vi "setAttributeByName.vi"(8 "error in (no error)":errorcluster, 9 "attributeValue":string, 10 "attributeName":string, 11 "xmlNode in":refnum<class "xmlNode.lvclass">) -> (0 "error out":errorcluster, 3 "xmlNode out":refnum<class "xmlNode.lvclass">)   [LabVIEW 2011, in "Tools.lvlib" / "xml.lvlib" / "xmlNode.lvclass"]
uses:
  xmlNode.lvclass
  xmlNode.lvclass/xmlNode.ctl
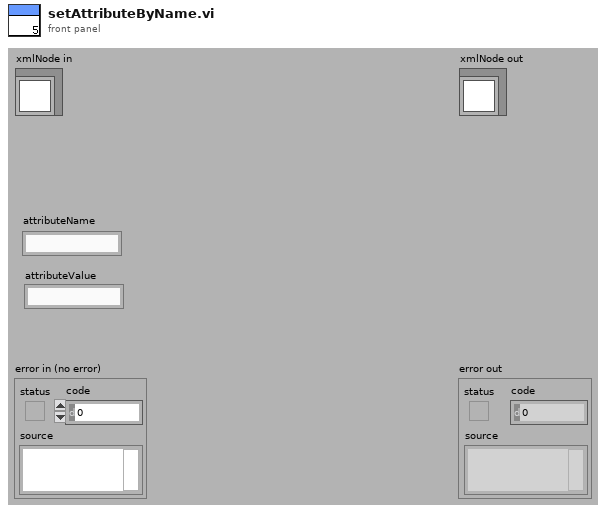
[diagram p1: front panel]
types:
  T1 = cluster{"attribute type":string, "attribute string":string}
  T2 = cluster{"attribute type":string, "attribute string":string}[]
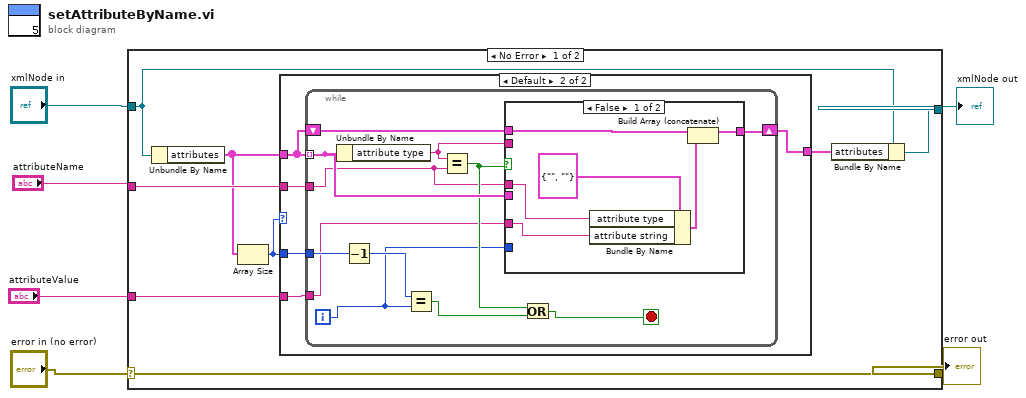
[diagram p0: block diagram]
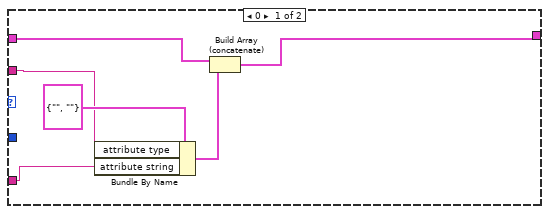
[diagram p2: hidden frame]
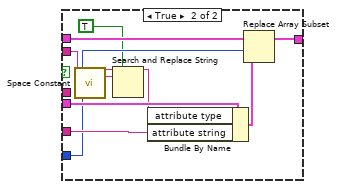
[diagram p3: hidden frame]
diagram:
  n1 = case shown="No Error" "error in (no error)" {
    selector: "error in (no error)" -> [w14 w55]
    tunnel: [w14 w55] -> w4
    tunnel: [w7 w54] -> w3
    tunnel: "xmlNode in" -> [w9 w54]
    tunnel: "attributeName" -> [w13 _]
    tunnel: "attributeValue" -> [w10 _]
    frame No Error {
      n2 = Unbundle By Name(w9) -> ("attributes"=w12:T2)
      n3 = Array Size(array=w12) -> (size(s)=w11:i32)
      n4 = case shown="Default" w11 {
        tunnel: w13 -> [w18 w25]
        tunnel: w12 -> [w16 w21]
        tunnel: w11 -> [_ w24]
        tunnel: [w15 w23] -> w8
        tunnel: w10 -> [w19 w22]
        frame 0 {
          n5 = Bundle By Name(cluster=T1 {"attribute type"="", "attribute string"=""} ("attribute"), "attribute type"=w18, "attribute string"=w19) -> (w17:T1)
          n6 = Build Array (concatenate)(w16, w17) -> (w15:T2)
        }
        frame Default {
          n7 = while {
            tunnel: w21 -> [w37] mode=indexing
            tunnel: w25 -> [w26]
            tunnel: w24 -> [w35]
            tunnel: w22 -> [w30]
            shift-right: [w28] -> w23
            shift-left: w21 -> [w29]
            i -> [w27]
            stop <- w32 stop-if-true
            n8 = Unbundle By Name(w37) -> ("attribute type"=w31:string)
            n9 = Decrement(x=w35) -> (x-1=w34:i32)
            n10 = Equal?(x=w34, y=w27) -> (x = y?=w33:bool)
            n11 = Equal?(x=w31, y=w26) -> (x = y?=w36:bool)
            n12 = case shown="False" w36 {
              tunnel: w37 -> [_ w53]
              tunnel: w31 -> [_ w47]
              tunnel: w30 -> [w39 w52]
              tunnel: w29 -> [w43 w51]
              tunnel: [w42 w50] -> w28
              tunnel: w27 -> [_ w48]
              tunnel: w26 -> [w40 _]
              frame False {
                n13 = Bundle By Name(cluster=T1 {"attribute type"="", "attribute string"=""} ("attribute"), "attribute type"=w40, "attribute string"=w39) -> (w38:T1)
                n14 = Build Array (concatenate)(w43, w38) -> (w42:T2)
              }
              frame True {
                n15 = call <vilib>:"Space Constant.vi"() -> ("String"=w44:string)
                n16 = Search and Replace String(replace all?=TRUE, input string=w47, search string=w44) -> (result string=w46:string)  [unwired: 5 in, 3 out]
                n17 = Bundle By Name(cluster=w53, "attribute type"=w46, "attribute string"=w52) -> (w49:T1)
                n18 = Replace Array Subset(array=w51, new element=w49, index=w48) -> (w50:T2)
              }
            }
            n19 = Or(x=w36, y=w33) -> (x .or. y?=w32:bool)
          }
        }
      }
      n20 = Bundle By Name(cluster=w9, "attributes"=w8) -> (w7:refnum<class "xmlNode.lvclass">)
    }
    frame Error {
    }
  }
  "error out" <- w4
  "xmlNode out" <- w3
